vi "anglestovector.vi"(8 "R":dbl=1.0, 10 "phi":dbl, 11 "theta":dbl) -> (1 "B":dbl[](array[numeric])=[0.1411200080598672, 0.0, -0.9899924966004454])   [LabVIEW 2018]
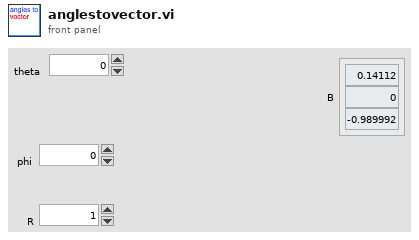
[diagram p1: front panel]
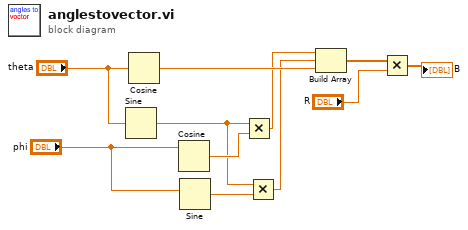
[diagram p0: block diagram]
diagram:
  n1 = Sine(x="theta") -> (sin(x)=w3:dbl)
  n2 = Cosine(x="theta") -> (cos(x)=w8:dbl)
  n3 = Cosine(x="phi") -> (cos(x)=w5:dbl)
  n4 = Sine(x="phi") -> (sin(x)=w2:dbl)
  n5 = Multiply(x=w3, y=w5) -> (x*y=w4:dbl)
  n6 = Multiply(x=w3, y=w2) -> (x*y=w1:dbl)
  n7 = Build Array(w4, w1, w8) -> (w11:dbl[])
  n8 = Multiply(x=w11, y="R") -> (x*y=→"B":dbl[])
